vi "Exercise4.3-Pre-Lab3.vi"() -> ()   [LabVIEW 2013]
panel:
  in  "Lower Cut-Off":dbl=100.0
  out "Waveform Graph 2":dynamicdata(graph)=[{"t0"=timestamp(4.6744537353515625 s since 1904-01-01), "dt"=0.0001, "Y"=array[1000 elements], "attributes"=variant("NI_ChannelName"=variant(string "Sine"), "NI_ExpIsRelativeTime"=variant(bool TRUE), "NI_ExpStartTimeStamp"=variant(timestamp timestamp(3695351012.694714 s since 1904-01-01)), "NI_ExpTimeStamp"=variant(timestamp timestamp(3695351017.369168 s since 1904-01-01)), "NI_ExpXDimension"=variant(string "t"))}]
  in  "stop":bool
  out "Waveform Graph":dynamicdata(graph)=[{"t0"=timestamp(4.667473793029785 s since 1904-01-01), "dt"=0.0001, "Y"=array[1000 elements], "attributes"=variant("NI_ChannelName"=variant(string "Sine (Filtered)"), "NI_ExpIsRelativeTime"=variant(bool TRUE), "NI_ExpStartTimeStamp"=variant(timestamp timestamp(3695351012.694714 s since 1904-01-01)), "NI_ExpTimeStamp"=variant(timestamp timestamp(3695351017.362188 s since 1904-01-01)), "NI_ExpXDimension"=variant(string "t"), "NI_OriginalChannelName"=variant(string "Sine"))}]
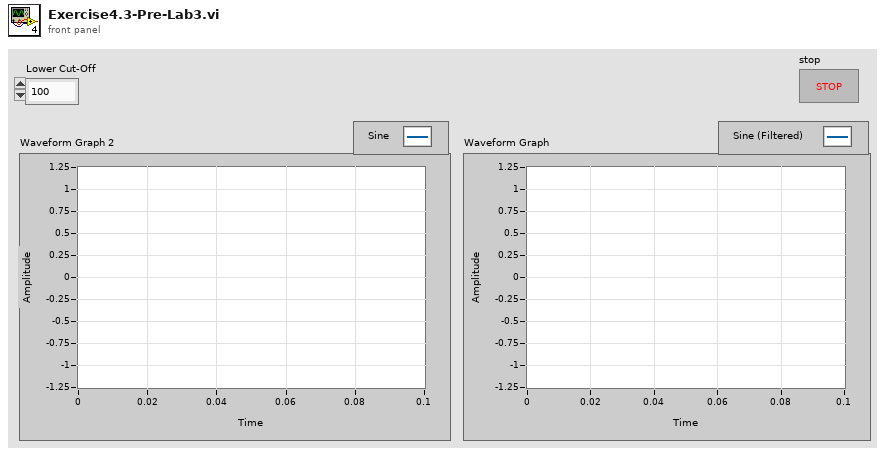
[diagram p1: front panel]
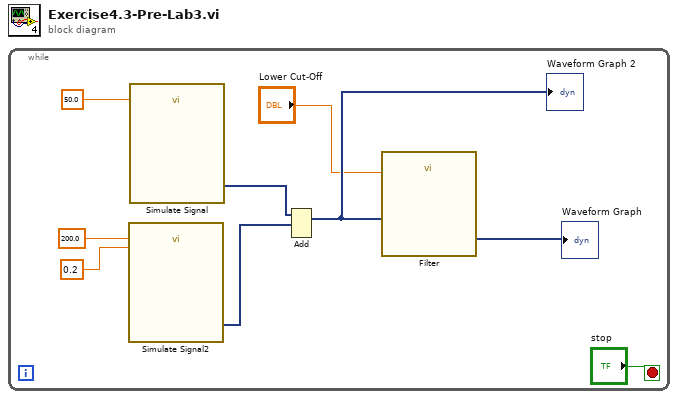
[diagram p0: block diagram]
diagram:
  n1 = while {
    stop <- "stop" stop-if-true
    n2 = call "Simulate Signal2"("Frequency"=200.0, "Amplitude"=0.2) -> ("Sine"=w6:dynamicdata)  [unwired: 12 in, 1 out]
    n3 = call "Simulate Signal"("Frequency"=50.0) -> ("Sine"=w7:dynamicdata)  [unwired: 13 in, 1 out]
    n4 = Add(1:w6, 2:w7) -> (0:w3:dynamicdata)  [unwired: 1 in, 1 out]
    "Waveform Graph 2" <- w3
    n5 = call "Filter"("Lower Cut-Off"="Lower Cut-Off", "Signal"=w3) -> ("Filtered Signal"=→"Waveform Graph":dynamicdata)  [unwired: 8 in, 1 out]
  }
